vi "Untitled 4.vi"() -> ()   [LabVIEW 2016]
panel:
  out "NaN/Path/Refnum? 4":bool
  out "NaN/Path/Refnum? 3":bool
  out "NaN/Path/Refnum? 2":bool
  out "NaN/Path/Refnum?":bool
  out "error out 2":errorcluster
  out "data out":string
  out "error out":errorcluster
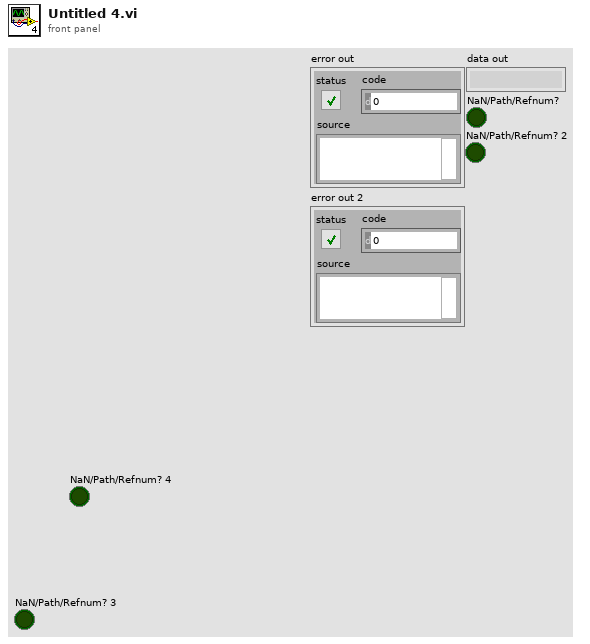
[diagram p1: front panel]
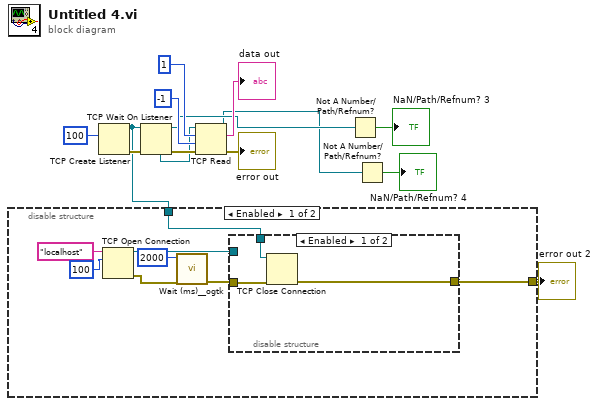
[diagram p0: block diagram]
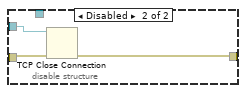
[diagram p2: hidden frame]
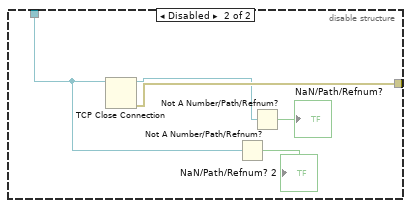
[diagram p3: hidden frame]
diagram:
  n1 = TCP Create Listener(10:u16 100 ("port")) -> (0:w14:errorcluster, 3:w1:refnum<k5>)  [unwired: 4 in, 1 out]
  n2 = disable-structure shown="Enabled" {
    disable-tunnel: [w16 w33] -> w7
    disable-tunnel: w1 -> [w15 w32]
    frame Enabled {
      n3 = TCP Open Connection(address="localhost", remote port or service name=u16 100) -> (connection ID=w21:refnum<k5>, error out=w19:errorcluster)  [unwired: 3 in]
      n4 = call <userlib>:"Wait (ms)__ogtk.vi"("error in (no error)"=w19, "milliseconds to wait"=u32 2000) -> ("error out"=w18:errorcluster)  [unwired: 8 in, 1 out]
      n5 = disable-structure shown="Enabled" {
        disable-tunnel: w21 -> [_ w28]
        disable-tunnel: w18 -> [w25 w27]
        disable-tunnel: w15 -> [w24 _]
        disable-tunnel: [w23 w26] -> w16
        frame Enabled {
          n6 = TCP Close Connection(connection ID=w24, error in (no error)=w25) -> (error out=w23:errorcluster)  [unwired: 1 in, 1 out]
        }
        frame Disabled {
          n7 = TCP Close Connection(connection ID=w28, error in (no error)=w27) -> (error out=w26:errorcluster)  [unwired: 1 in, 1 out]
        }
      }
    }
    frame Disabled {
      n8 = TCP Close Connection(connection ID=w32) -> (connection ID out=w31:refnum<k5>, error out=w33:errorcluster)  [unwired: 2 in]
      n9 = Not A Number/Path/Refnum?(number/path/refnum=w32) -> (NaN/Path/Refnum?=→"NaN/Path/Refnum? 2":bool)
      n10 = Not A Number/Path/Refnum?(number/path/refnum=w31) -> (NaN/Path/Refnum?=→"NaN/Path/Refnum?":bool)
    }
  }
  "error out 2" <- w7
  n11 = TCP Wait On Listener(8:w14, 11:w1) -> (0:w12:errorcluster, 3:w5:refnum<k5>, 4:w2:refnum<k5>)  [unwired: 2 in, 2 out]
  n12 = TCP Read(connection ID=w2, bytes to read=1, error in (no error)=w12, 9:-1 ("timeout ms (25000)")) -> (connection ID out=w3:refnum<k5>, data out=→"data out":string, error out=→"error out":errorcluster)  [unwired: 1 in]
  n13 = Not A Number/Path/Refnum?(number/path/refnum=w5) -> (NaN/Path/Refnum?=→"NaN/Path/Refnum? 3":bool)
  n14 = Not A Number/Path/Refnum?(number/path/refnum=w3) -> (NaN/Path/Refnum?=→"NaN/Path/Refnum? 4":bool)
